vi "test BC Only.vi"(8 "error in":errorcluster, 11 "TestCase in":refnum<class "Create Execution Unit.lvclass">) -> (0 "error out":errorcluster, 3 "TestCase out":refnum<class "Create Execution Unit.lvclass">)   [LabVIEW 2023, in "Create Execution Unit.lvclass"]
uses:
  Create Execution Unit.lvclass
  C:/Program Files/National Instruments/LabVIEW 2023/vi.lib/NI/VeriStand Custom Device Testing Tools/VeriStandScriptingTestCase/VeriStandScriptingTestCase.lvclass
  Engine/Implementation/Execution Unit Factory/Execution Unit Factory.lvclass
  Shared/Address.ctl
  Engine/Implementation/Rx Execution Unit/Rx Execution Unit.lvclass
  Engine/Custom Device/Logging Configuration.ctl
  Shared/Data Word Format.ctl
  Shared/Device Parameters.ctl
  Shared/Initialization Method.ctl
  Engine/Implementation/Tx Execution Unit/Tx Execution Unit.lvclass
  Engine/Implementation/Address Based Execution Unit/Address Based Execution Unit.lvclass
  <vilib>/NI/VeriStand Custom Device Testing Tools/VeriStandScriptingTestCase/VeriStandScriptingTestCase.lvclass/VeriStandScriptingTestCase.ctl
  Engine/Implementation/Tx Execution Unit/Tx Execution Unit.lvclass/Tx Execution Unit.ctl
  Engine/Implementation/Rx Execution Unit/Rx Execution Unit.lvclass/Rx Execution Unit.ctl
  <vilib>/NI/VeriStand Custom Device Testing Tools/VeriStandScriptingTestCase/Read Target.vi
  Engine/Implementation/Shared Resources/Shared Resources.lvclass
  C:/dev/niveristand-ballard-milStd1553-custom-device/Source/Custom Device Support/Engine/Interfaces/Shared Resources/Shared Resources.lvclass
  NationalInstruments.VeriStand.SystemDefinitionAPI
  Create Execution Unit.lvclass/Create Execution Unit.ctl
  <vilib>/addons/_JKI Toolkits/VI Tester/TestCase.llb/TestCase.lvclass
  Scripting/Ballard MIL-STD-1553 Scripting.lvlib
  Engine/Custom Device/Custom Device.lvlib
  C:/Program Files/National Instruments/LabVIEW 2023/vi.lib/addons/_JKI Toolkits/VI Tester/TestCase.llb/TestCase.lvclass
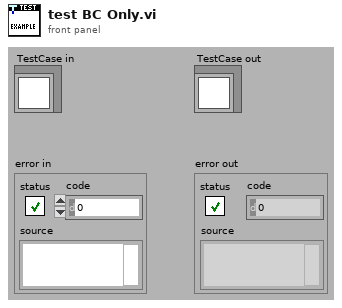
[diagram p1: front panel]
types:
  T1 = typedef "Device Parameters.ctl" = cluster{"initialization method":T2, "card number":i32, "PXI slot number":i32, "core number":i32}
  T2 = typedef "Initialization Method.ctl" = enum16{"PXI Slot Number", "Card Number"}
  T3 = typedef "Ballard MIL-STD-1553 Engine Support.lvlib/Custom Device.lvlib/Logging Configuration.ctl" = cluster{"configured":bool, "directory":string, "file name":string, "timestamp file name":bool, "data word format":T4}
  T4 = typedef "Data Word Format.ctl" = string
  T5 = typedef "Address.ctl" = u16
  T6 = cluster{"Hardware File":path, "Parameters File":path}
  T7 = typedef "Custom Device API.lvlib/Custom Device Item Ref.ctl" = u64
  T8 = typedef "1553 Channel.ctl" = cluster{"HW channel":u16, "bus controller":cluster{"simulated?":bool, "name":string}, "terminal addresses":T5[], "terminal names":string[], "acyclic frame names":string[], "messages":T9[]}
  T9 = typedef "Message Definition.ctl" = cluster{"name":string, "message type":T10, "endpoint Tx":T11, "endpoint Rx":T11, "create timestamp channel":bool, "mode code":u16, "number of words":u16, "parameters":cluster{"name":string, "default value":dbl, "unit":string, "parameter definition":T12}[]}
  T10 = typedef "Message Type.ctl" = string
  T11 = typedef "Terminal Endpoint.ctl" = cluster{"terminal address":T5, "subaddress":T5}
  T12 = typedef "Parameter Definition.ctl" = cluster{"start index":i32, "size (bits)":i32, "encoding":enum16{"BNR", "BCD", "Discrete"}, "signed":bool, "multiplier":dbl, "offset":dbl}
  T13 = typedef "Ballard MIL-STD-1553 Engine Support.lvlib/Interfaces.lvlib/Execution Unit Information.ctl" = cluster{"Execution Unit":refnum<class "Execution Unit.lvclass">, "Incoming Channels":T7[], "Outgoing Channels":T7[], "ReadWrite Channels":T7[]}
  T14 = typedef "Map of Messages to Value Indexes.ctl" = map{T15, T16}
  T15 = typedef "Message Map Key.ctl" = cluster{"HW channel":u16, "terminal address":u16, "subaddress":u16, "mode code":u16}
  T16 = typedef "Ballard MIL-STD-1553 Engine Support.lvlib/Implementation.lvlib/Rx Execution Unit.lvclass/Message Map Value.ctl" = cluster{"value indexes":i32[], "message":T9, "Tx status count":i32, "Rx status count":i32}
  T17 = typedef "Tx Write Info.ctl" = cluster{"transfer handle":u64, "value index":i32}
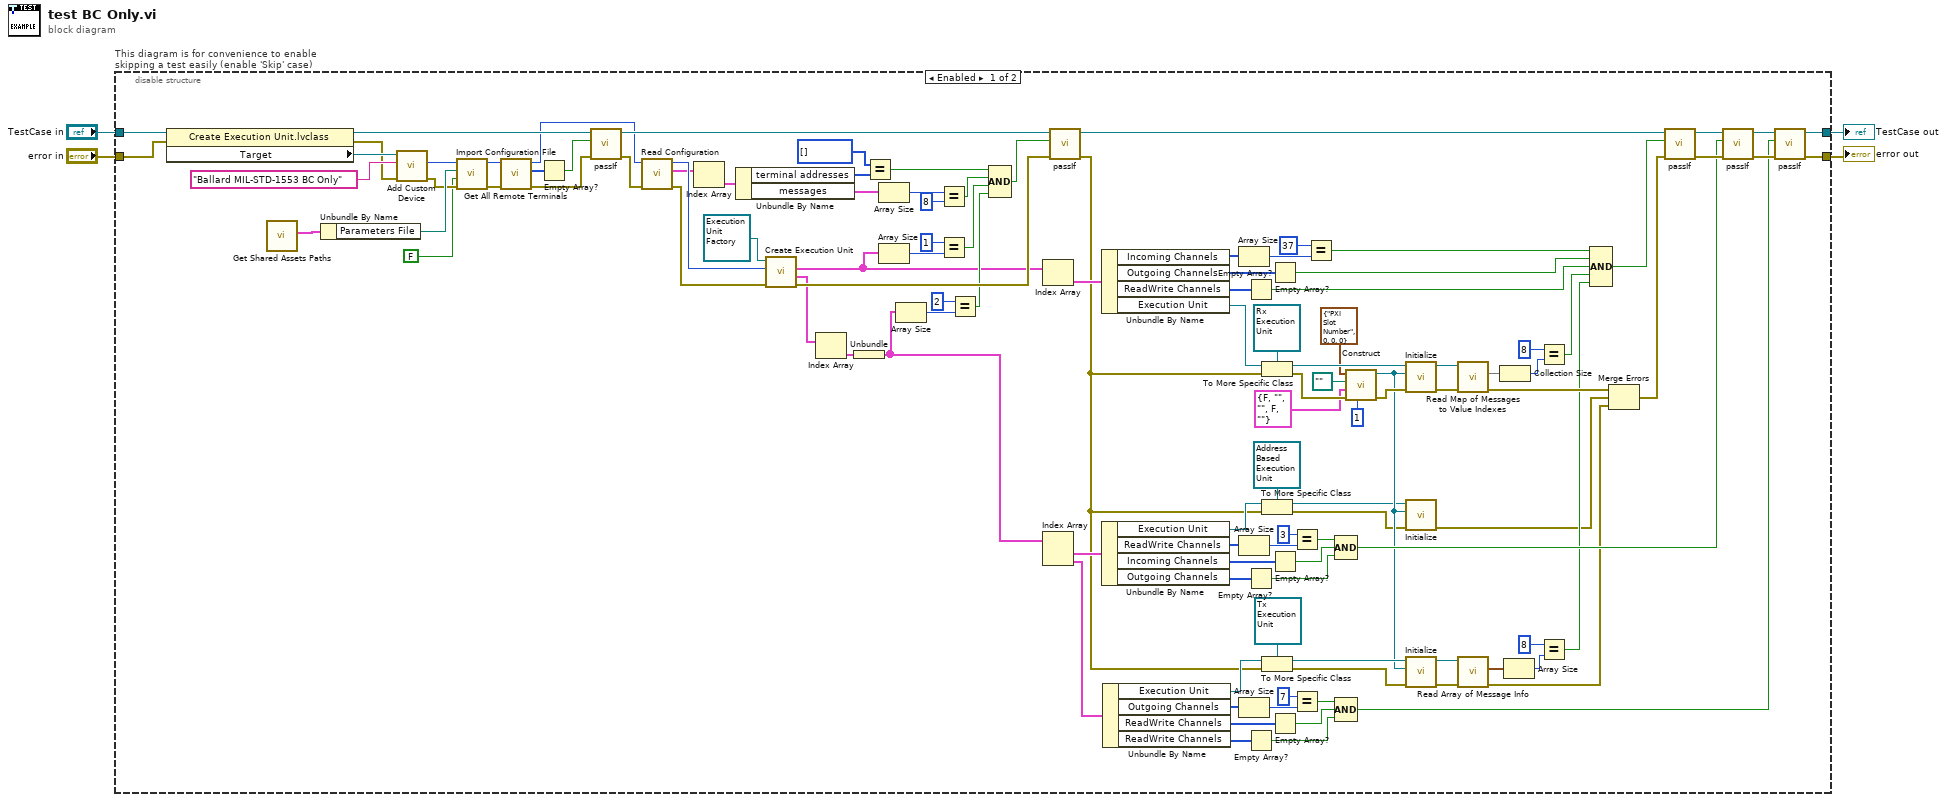
[diagram p0: block diagram]
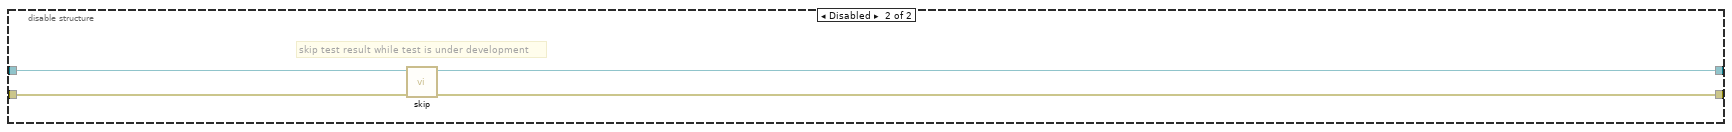
[diagram p2: hidden frame]
diagram:
  n1 = disable-structure "This diagram is for convenience to enable skipping a test easily (enable 'Skip' case)" shown="Enabled" {
    disable-tunnel: "TestCase in" -> [w114 w123]
    disable-tunnel: [w49 w121] -> w1
    disable-tunnel: [w54 w122] -> w3
    disable-tunnel: "error in" -> [w118 w120]
    frame Enabled {
      n2 = property class="Create Execution Unit.lvclass"(reference=w114, error in=w118) -> (reference out=w119:refnum<class "Create Execution Unit.lvclass">, error out=w115:errorcluster, "Target"=w116:refnum<k24>)
      n3 = call "Get Shared Assets Paths.vi"() -> ("BC Only"=w15:T6)  [unwired: 9 in, 2 out]
      n4 = Unbundle By Name(w15) -> ("Parameters File"=w14:path)
      n5 = call "Add Custom Device.vi"("error in"=w115, "name"="Ballard MIL-STD-1553 BC Only", "target in"=w116) -> ("error out"=w12:errorcluster, "Ballard MIL-STD 1553 custom device"=w13:T7)  [unwired: 6 in, 1 out]
      n6 = call "Import Configuration File.vi"("error in"=w12, "create Tx/Rx folders for subaddresses?"=FALSE, "parameters configuration file path"=w14, "Ballard MIL-STD 1553 custom device in"=w13) -> ("error out"=w10:errorcluster, "Ballard MIL-STD 1553 custom device out"=w11:T7)  [unwired: 6 in]
      n7 = call "Get All Remote Terminals.vi"("error in"=w10, "port in"=w11) -> ("error out"=w112:errorcluster, "remote terminals"=w113:T7[], "port out"=w90:T7)  [unwired: 7 in]
      n8 = Empty Array?(array=w113) -> (empty?=w111:bool)
      n9 = call-dynamic "passIf.vi"("error in (no error)"=w112, "pass"=w111, "TestCase in"=w119) -> ("error out"=w105:errorcluster, "TestCase out"=w94:refnum<class "Create Execution Unit.lvclass">)  [unwired: 7 in]
      n10 = call "Read Configuration.vi"("error in"=w105, "Ballard MIL-STD 1553 custom device in"=w90) -> ("error out"=w104:errorcluster, "1553 channels"=w102:T8[], "Ballard MIL-STD 1553 custom device out"=w103:T7)  [unwired: 7 in]
      n11 = Index Array(array=w102) -> (element=w101:T8)  [unwired: 1 in]
      n12 = Unbundle By Name(w101) -> ("terminal addresses"=w100:T5[], "messages"=w98:T9[])
      n13 = call-dynamic "Create Execution Unit.vi"("error in"=w104, "Item Ref"=w103, "Execution Unit Factory Implementation in"=refnum<class "Execution Unit Factory.lvclass"> refnum) -> ("error out"=w93:errorcluster, "Asynchronous Execution Units"=w86:cluster{"Grouped Execution Units":T13[]}[], "Inline Execution Units"=w87:T13[])  [unwired: 5 in, 1 out]
      n14 = Index Array(array=w86) -> (element=w9:cluster{"Grouped Execution Units":T13[]})  [unwired: 1 in]
      n15 = Unbundle(w9) -> ("Grouped Execution Units"=w8:T13[])
      n16 = Equal?(x=T5[] [] ("terminal addresses"), y=w100) -> (x = y?=w91:bool)
      n17 = Array Size(array=w98) -> (size(s)=w96:i32)
      n18 = Array Size(array=w87) -> (size(s)=w109:i32)
      n19 = Array Size(array=w8) -> (size(s)=w108:i32)
      n20 = Equal?(x=w96, y=8 ("x")) -> (x = y?=w95:bool)
      n21 = Equal?(x=1, y=w109) -> (x = y?=w89:bool)
      n22 = Equal?(x=2, y=w108) -> (x = y?=w88:bool)
      n23 = Compound Arithmetic op=AND(w91, w95, w89, w88) -> (w92:bool)
      n24 = Index Array(array=w87) -> (element=w85:T13)  [unwired: 1 in]
      n25 = Index Array(array=w8) -> (element #1=w84:T13, element #2=w83:T13)  [unwired: 2 in]
      n26 = call-dynamic "passIf.vi"("error in (no error)"=w93, "pass"=w92, "TestCase in"=w94) -> ("error out"=w20:errorcluster, "TestCase out"=w81:refnum<class "Create Execution Unit.lvclass">)  [unwired: 7 in]
      n27 = Unbundle By Name(w85) -> ("Incoming Channels"=w82:T7[], "Outgoing Channels"=w68:T7[], "ReadWrite Channels"=w67:T7[], "Execution Unit"=w71:refnum<class "Execution Unit.lvclass">)
      n28 = Unbundle By Name(w84) -> ("Execution Unit"=w22:refnum<class "Execution Unit.lvclass">, "ReadWrite Channels"=w60:T7[], "Incoming Channels"=w59:T7[], "Outgoing Channels"=w58:T7[])
      n29 = Unbundle By Name(w83) -> ("Execution Unit"=w32:refnum<class "Execution Unit.lvclass">, "Outgoing Channels"=w46:T7[], "ReadWrite Channels"=w45:T7[], "ReadWrite Channels"=w44:T7[])
      n30 = Array Size(array=w82) -> (size(s)=w69:i32)
      n31 = Array Size(array=w60) -> (size(s)=w62:i32)
      n32 = Array Size(array=w46) -> (size(s)=w47:i32)
      n33 = Empty Array?(array=w67) -> (empty?=w64:bool)
      n34 = Empty Array?(array=w58) -> (empty?=w55:bool)
      n35 = Empty Array?(array=w44) -> (empty?=w41:bool)
      n36 = To More Specific Class(target class=refnum<class "Rx Execution Unit.lvclass"> refnum ("Rx execution unit in"), reference=w71, error in=w20) -> (specific class reference=w78:refnum<class "Rx Execution Unit.lvclass">, error out=w76:errorcluster)
      n37 = To More Specific Class(target class=refnum<class "Address Based Execution Unit.lvclass"> refnum ("Address Based Execution Unit Implementation in"), reference=w22, error in=w20) -> (specific class reference=w19:refnum<class "Address Based Execution Unit.lvclass">, error out=w18:errorcluster)
      n38 = To More Specific Class(target class=refnum<class "Tx Execution Unit.lvclass"> refnum ("Tx Execution Unit Implementation in"), reference=w32, error in=w20) -> (specific class reference=w31:refnum<class "Tx Execution Unit.lvclass">, error out=w30:errorcluster)
      n39 = Empty Array?(array=w68) -> (empty?=w65:bool)
      n40 = Empty Array?(array=w59) -> (empty?=w56:bool)
      n41 = Empty Array?(array=w45) -> (empty?=w42:bool)
      n42 = Equal?(x=3 ("size(s)"), y=w62) -> (x = y?=w57:bool)
      n43 = Equal?(x=7 ("size(s)"), y=w47) -> (x = y?=w43:bool)
      n44 = Equal?(x=37 ("size(s)"), y=w69) -> (x = y?=w66:bool)
      n45 = Compound Arithmetic op=AND(w57, w56, w55) -> (w40:bool)
      n46 = Compound Arithmetic op=AND(w43, w42, w41) -> (w39:bool)
      n47 = call "Construct.vi"("number of ports"=1, "error in"=w76, "logging configuration"=T3 {"configured"=FALSE, "directory"="", "file name"="", "timestamp file name"=FALSE, "data word format"=""}, "hardware config file"=path "", "device parameters"=T1 {"initialization method"=enum."PXI Slot Number", "card number"=0, "PXI slot number"=0, "core number"=0}) -> ("error out"=w75:errorcluster, "Ballard 1553 shared resources"=w23:refnum<class "Shared Resources.lvclass">)  [unwired: 5 in]
      n48 = call-dynamic "Initialize.vi"("error in"=w75, "shared resources"=w23, "Rx Execution Unit Implementation in"=w78) -> ("error out"=w16:errorcluster, "Rx Execution Unit Implementation out"=w79:refnum<class "Rx Execution Unit.lvclass">)  [unwired: 7 in]
      n49 = call-dynamic "Initialize.vi"("error in"=w18, "shared resources"=w23, "Address Based Execution Unit Implementation in"=w19) -> ("error out"=w17:errorcluster)  [unwired: 7 in, 1 out]
      n50 = call-dynamic "Initialize.vi"("error in"=w30, "shared resources"=w23, "Tx Execution Unit Implementation in"=w31) -> ("error out"=w29:errorcluster, "Tx Execution Unit Implementation out"=w34:refnum<class "Tx Execution Unit.lvclass">)  [unwired: 7 in]
      n51 = call "Read Map of Messages to Value Indexes.vi"("error in"=w16, "Rx execution unit in"=w79) -> ("error out"=w27:errorcluster, "map of messages to value indexes"=w37:T14)  [unwired: 7 in, 1 out]
      n52 = call "Read Array of Message Info.vi"("error in"=w29, "Tx execution unit in"=w34) -> ("error out"=w28:errorcluster, "array of message info"=w6:T17[])  [unwired: 7 in, 1 out]
      n53 = Collection Size(1:w37) -> (0:w36:i32)
      n54 = Array Size(array=w6) -> (size(s)=w7:i32)
      n55 = Equal?(x=8 ("size(s)"), y=w36) -> (x = y?=w35:bool)
      n56 = Equal?(x=8 ("size(s)"), y=w7) -> (x = y?=w24:bool)
      n57 = Compound Arithmetic op=AND(w66, w65, w64, w35, w24) -> (w63:bool)
      n58 = Merge Errors(w27, w17, w28) -> (w26:errorcluster)
      n59 = call-dynamic "passIf.vi"("error in (no error)"=w26, "pass"=w63, "TestCase in"=w81) -> ("error out"=w52:errorcluster, "TestCase out"=w53:refnum<class "Create Execution Unit.lvclass">)  [unwired: 7 in]
      n60 = call-dynamic "passIf.vi"("error in (no error)"=w52, "pass"=w40, "TestCase in"=w53) -> ("error out"=w50:errorcluster, "TestCase out"=w51:refnum<class "Create Execution Unit.lvclass">)  [unwired: 7 in]
      n61 = call-dynamic "passIf.vi"("error in (no error)"=w50, "pass"=w39, "TestCase in"=w51) -> ("error out"=w54:errorcluster, "TestCase out"=w49:refnum<class "Create Execution Unit.lvclass">)  [unwired: 7 in]
    }
    frame Disabled {
      # "skip test result while test is under development"
      n62 = call <vilib>:"skip.vi"("error in (no error)"=w120, "TestCase in"=w123) -> ("error out"=w122:errorcluster, "TestCase out"=w121:refnum<class "Create Execution Unit.lvclass">)  [unwired: 8 in]
    }
  }
  "error out" <- w3
  "TestCase out" <- w1
